vi "Enabled CRef.vi"() -> (6 "Enabled: CRef":T1)   [LabVIEW 2010, in "FTC.lvlib"]
uses:
  FTC.lvlib
  CLIB/CRef/Interface/CRef Boolean.llb/Boolean CReference.ctl
  CLIB/CRef/CRef.lvlib
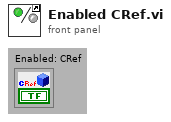
[diagram p1: front panel]
types:
  T1 = typedef "CRef.lvlib/Boolean CReference.ctl" = cluster{"Boolean CRef Address":u16, "Type":enum8{"Null", "Boolean", "U8", "I8", "U16", "I16", "U32", "I32", "U64", "I64", "Single", "Double", "Extended", "CSG", "CDB", "CXT", "Boolean(Def)"}}
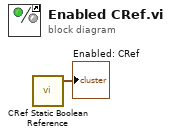
[diagram p0: block diagram]
diagram:
  n1 = call "CRef Static Boolean Reference.vi"() -> ("Boolean CReference"=→"Enabled: CRef":T1)  [unwired: 5 in]
